vi "fgv_imu_232.vi"(7 "cmd":enum16{"init", "read", "write", "close"}(ring), 8 "error in":errorcluster, 11 "write buff":string) -> (0 "error out":errorcluster, 2 "byte n":u32(graph), 3 "read_buffer":string)   [LabVIEW 2019]
uses:
  <vilib>/Instr/_visa.llb/VISA Configure Serial Port (Instr).vi
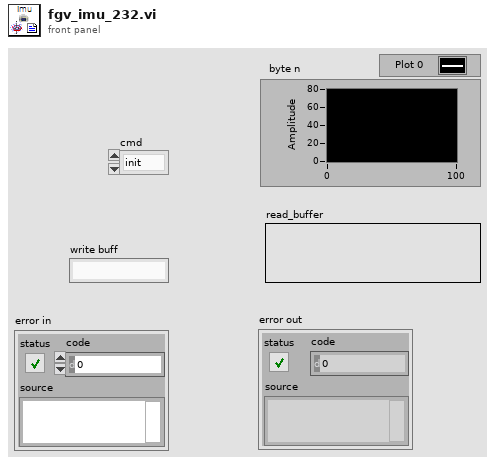
[diagram p1: front panel]
types:
  T1 = typedef "imu-cfg.ctl" = cluster{"Port":refnum<visa-resource-name>, "cmd":string, "rate":u32}
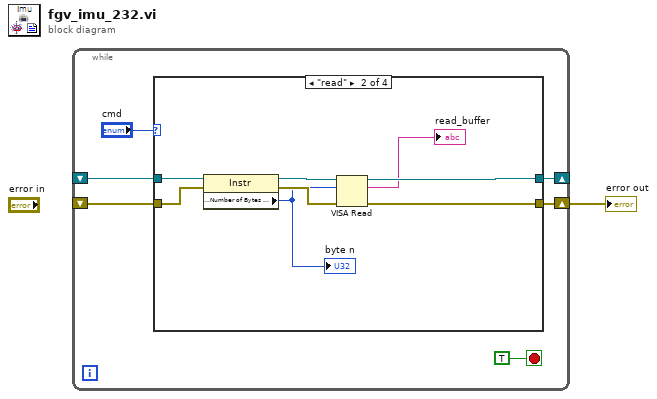
[diagram p0: block diagram]
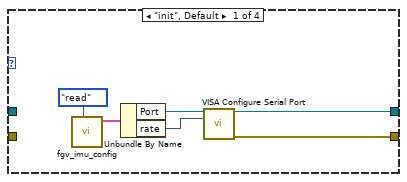
[diagram p2: hidden frame]
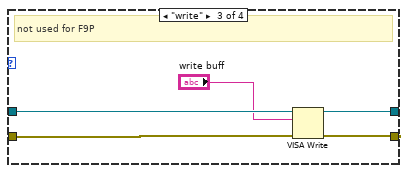
[diagram p3: hidden frame]
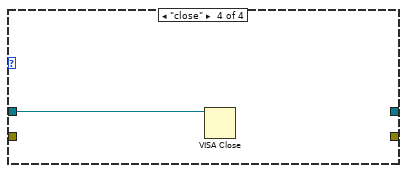
[diagram p4: hidden frame]
diagram:
  n1 = while {
    shift-right: [w5] -> _
    shift-left: _ -> [w3]
    shift-right: [w4] -> w1
    shift-left: _ -> [w2]
    stop <- TRUE stop-if-true
    n2 = case shown="\"read\"" "cmd" {
      tunnel: [w13 w19 w24 _] -> w5
      tunnel: [w12 w18 w23 _] -> w4
      tunnel: w3 -> [_ w21 w25 w27]
      tunnel: w2 -> [_ w16 w26 _]
      frame "init", Default {
        n3 = call "fgv_imu_config.vi"("cmd"=enum16{"read", "write"}."read") -> ("IMU cfg out"=w9:T1)  [unwired: 9 in, 1 out]
        n4 = Unbundle By Name(w9) -> ("Port"=w11:refnum<visa-resource-name>, "rate"=w10:u32)
        n5 = call-poly "VISA Configure Serial Port"("VISA resource name"=w11, "baud rate (9600)"=w10) -> ("VISA resource name out"=w13:refnum<visa-resource-name>, "error out"=w12:errorcluster)  [unwired: 12 in]
      }
      frame "read" {
        n6 = property class="Instr"(reference=w21, error in=w16) -> (reference out=w20:refnum<visa-resource-name>, error out=w17:errorcluster, "Serial Settings:Number of Bytes at Serial Port"=w14:u32)
        "byte n" <- w14
        n7 = VISA Read(VISA resource name=w20, byte count=w14, error in (no error)=w17) -> (VISA resource name out=w19:refnum<visa-resource-name>, read buffer=→"read_buffer":string, error out=w18:errorcluster)  [unwired: 1 out]
      }
      frame "write" {
        # "not used for F9P"
        n8 = VISA Write(VISA resource name=w25, write buffer="write buff", error in (no error)=w26) -> (VISA resource name out=w24:refnum<visa-resource-name>, error out=w23:errorcluster)  [unwired: 1 out]
      }
      frame "close" {
        n9 = VISA Close(VISA resource name=w27) -> ()  [unwired: 1 in, 1 out]
      }
    }
  }
  "error out" <- w1
